vi "DoManualJog.vi"(8 "Error In":errorcluster, 11 "MotorController in":refnum<class "MotorController.lvclass">) -> (0 "Error Out":errorcluster, 3 "MotorController out":refnum<class "MotorController.lvclass">)   [LabVIEW 2019]
uses:
  Axes_enum_typedef.ctl
  MotorController.lvclass
  DoManualJog_states_enum_typedef.ctl
panel:
  in  "Move":bool
  in  "Zero":bool
  in  "Done":bool
  in  "Position":i16
  in  "Axis":T1
  in  "Type of move":enum16{"Absolute Degrees", "Relative Step Jog"}(ring)
  # "Manual Jog"
  # "Use the controls below to manually move the machine in absolute or relative ways. Realtive movements loose position information!"
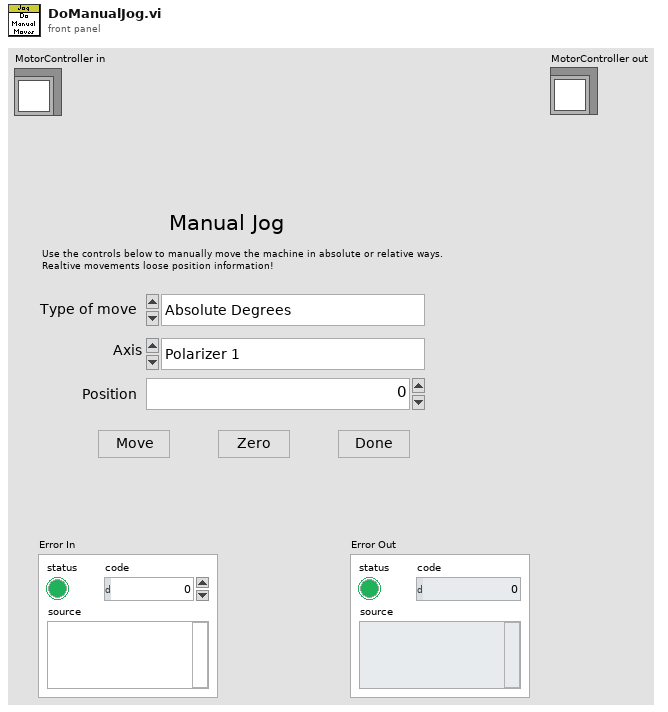
[diagram p1: front panel]
types:
  T1 = typedef "Axes_enum_typedef.ctl" = enum16{"Polarizer 1", "Polarizer 2", "Sample", "Stage"}
  T2 = typedef "DoManualJog_states_enum_typedef.ctl" = enum16{"Shutdown", "Zero", "Move", "Wait", "Initialize"}
  T3 = enum8{"Enabled", "Disabled", "Disabled and Grayed Out"}
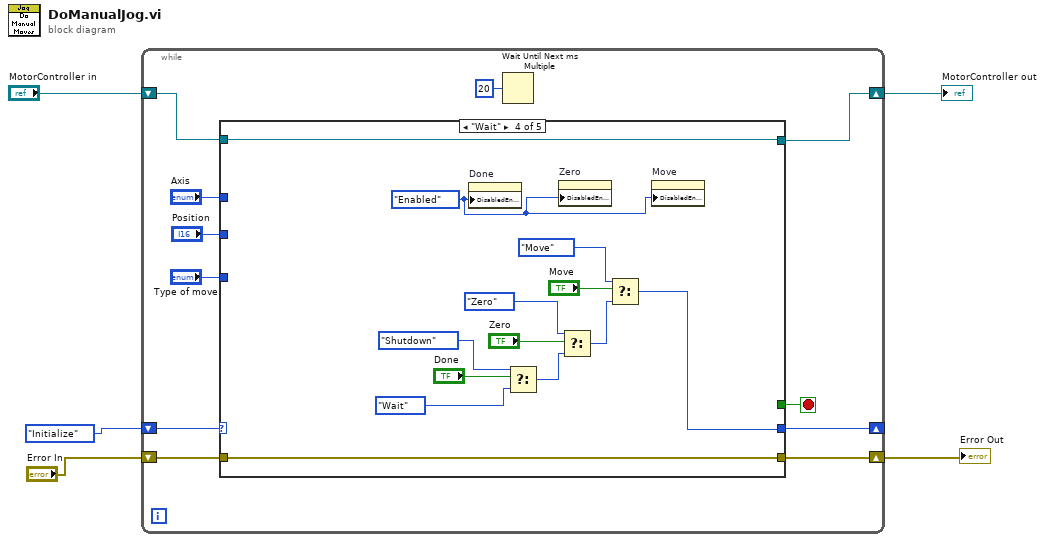
[diagram p0: block diagram]
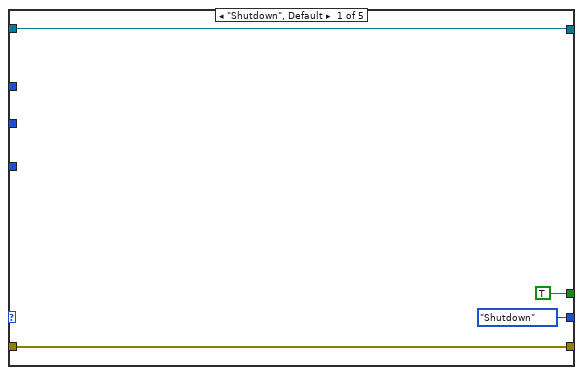
[diagram p2: hidden frame]
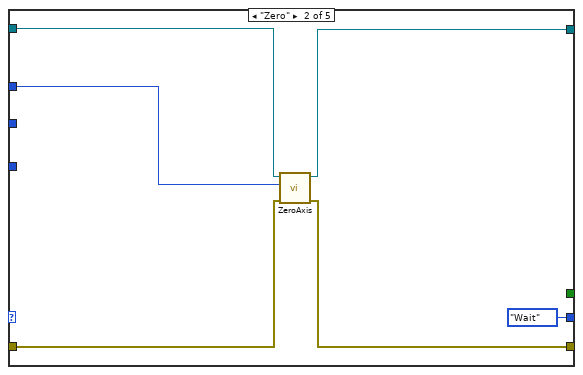
[diagram p3: hidden frame]
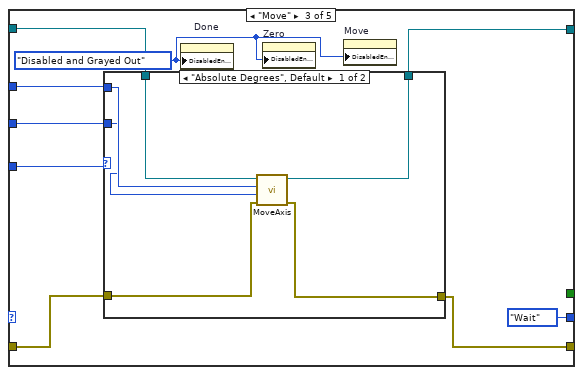
[diagram p4: hidden frame]
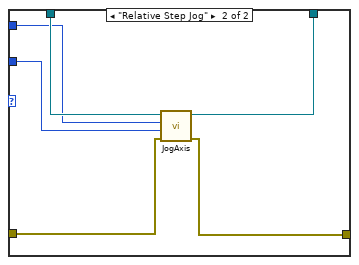
[diagram p5: hidden frame]
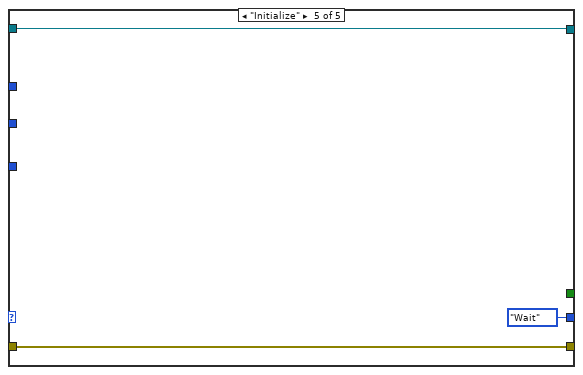
[diagram p6: hidden frame]
diagram:
  n1 = while {
    shift-right: [w13] -> _
    shift-left: DoManualJog_states_enum_typedef."Initialize" -> [w16]
    shift-right: [w12] -> w3
    shift-left: "Error In" -> [w15]
    shift-right: [w9] -> w1
    shift-left: "MotorController in" -> [w11]
    stop <- w6 stop-if-true
    n2 = case shown="\"Wait\"" w16 {
      tunnel: w15 -> [w18 w24 w32 w50 w61]
      tunnel: [DoManualJog_states_enum_typedef."Shutdown" DoManualJog_states_enum_typedef."Wait" DoManualJog_states_enum_typedef."Wait" w51 DoManualJog_states_enum_typedef."Wait"] -> w13
      tunnel: [w18 w23 w31 w50 w61] -> w12
      tunnel: w11 -> [w20 w26 w34 w49 w63]
      tunnel: "Type of move" -> [_ _ w35 _ _]
      tunnel: [w20 w25 w33 w49 w63] -> w9
      tunnel: "Axis" -> [_ w21 w30 _ _]
      tunnel: "Position" -> [_ _ w29 _ _]
      tunnel: [TRUE _ _ _ _] -> w6
      frame "Shutdown", Default {
      }
      frame "Zero" {
        n3 = call "ZeroAxis.vi"("error in (no error)"=w24, "Axis"=w21, "MotorController in"=w26) -> ("error out"=w23:errorcluster, "MotorController out"=w25:refnum<class "MotorController.lvclass">)  [unwired: 7 in]
      }
      frame "Move" {
        w27 = T3."Disabled and Grayed Out" ("Disabled")
        n4 = case shown="\"Absolute Degrees\", Default" w35 {
          tunnel: w34 -> [w41 w47]
          tunnel: [w40 w46] -> w33
          tunnel: w32 -> [w38 w45]
          tunnel: [w39 w44] -> w31
          tunnel: w30 -> [w37 w43]
          tunnel: w29 -> [w36 w42]
          frame "Absolute Degrees", Default {
            n5 = call "MoveAxis.vi"("error in (no error)"=w38, "Position"=w36, "Axis"=w37, "MotorController in"=w41) -> ("error out"=w39:errorcluster, "MotorController out"=w40:refnum<class "MotorController.lvclass">)  [unwired: 6 in]
          }
          frame "Relative Step Jog" {
            n6 = call "JogAxis.vi"("error in (no error)"=w45, "Steps"=w42, "Axis"=w43, "MotorController in"=w47) -> ("error out"=w44:errorcluster, "MotorController out"=w46:refnum<class "MotorController.lvclass">)  [unwired: 6 in]
          }
        }
        n7 = property on="Done" class="Bool"("DisabledEnum"=w27) -> ()  [unwired: 2 in, 2 out]
        n8 = property on="Zero" class="Bool"("DisabledEnum"=w27) -> ()  [unwired: 2 in, 2 out]
        n9 = property on="Move" class="Bool"("DisabledEnum"=w27) -> ()  [unwired: 2 in, 2 out]
      }
      frame "Wait" {
        w48 = T3."Enabled" ("Disabled")
        n10 = property on="Done" class="Bool"("DisabledEnum"=w48) -> ()  [unwired: 2 in, 2 out]
        n11 = Select(t=DoManualJog_states_enum_typedef."Shutdown", s="Done", f=DoManualJog_states_enum_typedef."Wait") -> (s? t:f=w52:T2)
        n12 = property on="Zero" class="Bool"("DisabledEnum"=w48) -> ()  [unwired: 2 in, 2 out]
        n13 = Select(t=DoManualJog_states_enum_typedef."Zero", s="Zero", f=w52) -> (s? t:f=w58:T2)
        n14 = Select(t=DoManualJog_states_enum_typedef."Move", s="Move", f=w58) -> (s? t:f=w51:T2)
        n15 = property on="Move" class="Bool"("DisabledEnum"=w48) -> ()  [unwired: 2 in, 2 out]
      }
      frame "Initialize" {
      }
    }
    n16 = Wait Until Next ms Multiple(millisecond multiple=u32 20) -> ()  [unwired: 1 out]
  }
  "Error Out" <- w3
  "MotorController out" <- w1
